vi "Main Avance.vi"() -> ()   [LabVIEW 2021]
uses:
  Class Selector.ctl
  Format Key Class/Format Key Class.lvclass
  Library.lvlib
panel:
  in  "Class":T1
  out "Value":string
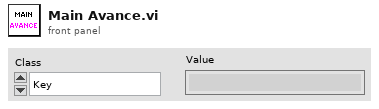
[diagram p1: front panel]
types:
  T1 = typedef "Library.lvlib/Class Selector.ctl" = enum16{"Key", "CSV"}
  T2 = map{string, refnum<class "Format Key Class.lvclass">}
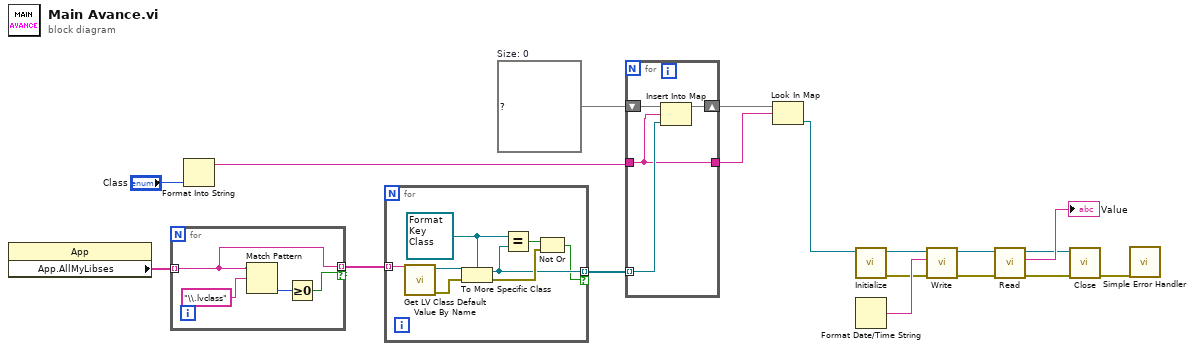
[diagram p0: block diagram]
diagram:
  w5 = T2 {}  # Size: 0
  n1 = property class="App"() -> ("App.AllMyLibses"=w9:string[])  [unwired: 2 in, 2 out]
  n2 = for {
    tunnel: w9 -> [w20] mode=indexing
    tunnel: [w20] -> w6 mode=indexing if=w22
    n3 = Match Pattern(string=w20, regular expression="\\.lvclass" ("search string/char (-)")) -> (offset past match=w21:i32)  [unwired: 1 in, 3 out]
    n4 = Greater Or Equal To 0?(x=w21) -> (x >= 0?=w22:bool)
  }
  n5 = Format Into String("Class") -> (resulting string=w7:string)  [unwired: 3 in, 1 out]
  n6 = for {
    tunnel: w6 -> [w30] mode=indexing
    tunnel: [w24] -> w4 mode=indexing if=w23
    w27 = refnum<class "Format Key Class.lvclass"> refnum ("Library.lvlib:Format Key Class")
    n7 = call <vilib>:"Get LV Class Default Value By Name.vi"("class name"=w30) -> ("error out"=w28:errorcluster, "object"=w29:refnum<class>)  [unwired: 9 in]
    n8 = To More Specific Class(target class=w27, reference=w29, error in=w28) -> (specific class reference=w24:refnum<class "Format Key Class.lvclass">, error out=w25:errorcluster)
    n9 = Equal?(x=w27, y=w24) -> (x = y?=w26:bool)
    n10 = Not Or(1:w25, 2:w26) -> (0:w23:bool)
  }
  n11 = for {
    shift-right: [w33] -> w3
    shift-left: w5 -> [w34]
    tunnel: w4 -> [w32] mode=indexing
    tunnel: w7 -> [w31]
    tunnel: [w31] -> w2
    n12 = Insert Into Map(map in=w34, key=w31, value=w32) -> (map out=w33:T2)  [unwired: 2 out]
  }
  n13 = Look In Map(map=w3, key=w2) -> (value=w1:refnum<class "Format Key Class.lvclass">)  [unwired: 1 in, 1 out]
  n14 = call-dynamic "Initialize.vi"("Format Key Class in"=w1) -> ("error out"=w11:errorcluster, "Format Key Class out"=w10:refnum<class "Format Key Class.lvclass">)  [unwired: 9 in]
  n15 = Format Date/Time String() -> (date/time string=w17:string)  [unwired: 3 in]
  n16 = call-dynamic "Write.vi"("error in (no error)"=w11, "Value"=w17, "Format Key Class in"=w10) -> ("error out"=w13:errorcluster, "Format Key Class out"=w12:refnum<class "Format Key Class.lvclass">)  [unwired: 7 in]
  n17 = call-dynamic "Read.vi"("error in (no error)"=w13, "Format Key Class in"=w12) -> ("error out"=w15:errorcluster, "Value"=→"Value":string, "Format Key Class out"=w14:refnum<class "Format Key Class.lvclass">)  [unwired: 7 in]
  n18 = call-dynamic "Close.vi"("error in (no error)"=w15, "Format Key Class in"=w14) -> ("error out"=w16:errorcluster)  [unwired: 8 in, 1 out]
  n19 = call <vilib>:"Simple Error Handler.vi"("error in (no error)"=w16) -> ()  [unwired: 4 in, 5 out]
